vi "Compare.vi"(8 "error in (no error)":errorcluster, 10 "Level":dbl, 11 "Color Strategy in":refnum<class "Color Strategy.lvclass">) -> (0 "error out":errorcluster, 2 "Color":u32(colorbox))   [LabVIEW 2021, in "Color Strategy.lvclass"]
uses:
  Color Strategy.lvclass
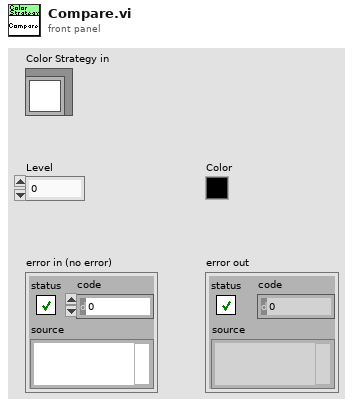
[diagram p1: front panel]
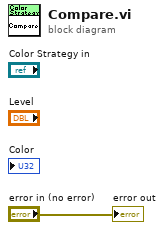
[diagram p0: block diagram]
diagram:
  "error out" <- "error in (no error)"
